vi "excel_read_data.vi"(8 "error in (no error)":errorcluster, 11 "Excel data":path) -> (0 "error out":errorcluster, 2 "wv_length_weight":dbl[](array[numeric]), 3 "wv_length_data":dbl[](array[numeric]))   [LabVIEW 2017]
uses:
  <vilib>/addons/_office/excel.llb/Excel Get Data ([dbl]).vi
  <vilib>/Utility/NIReport.llb/NI_report.lvclass
  <vilib>/Utility/NIReport.llb/Excel/NI_Excel.lvclass
  <vilib>/addons/_office/NI_ReportGenerationToolkit.lvlib
panel:
  out "wv_length and weight":dbl[][](array[numeric]) format="%.2f"
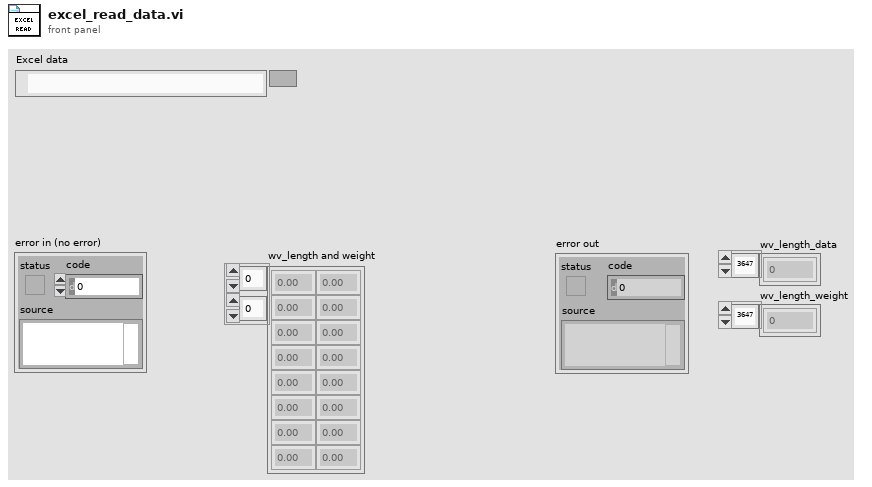
[diagram p1: front panel]
types:
  T1 = enum16{"Standard Report", "HTML", "Word", "Excel"}
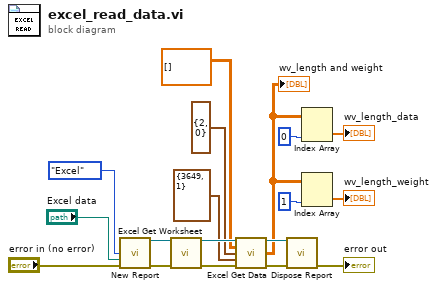
[diagram p0: block diagram]
diagram:
  n1 = call <vilib>:"New Report.vi"("report type"=T1."Excel", "template (empty)"="Excel data", "error in (no error)"="error in (no error)") -> ("report out"=w16:refnum<class "NI_report.lvclass">, "error out"=w15:errorcluster)  [unwired: 11 in]
  n2 = call <vilib>:"Excel Get Worksheet.vi"("report in"=w16, "error in (no error)"=w15) -> ("report out"=w13:refnum<class "NI_report.lvclass">, "error out"=w12:errorcluster)  [unwired: 12 in]
  n3 = call-poly <vilib>:"Excel Get Data.vi"("report in"=w13, "data type"=dbl[][] [], "start (-1, -1)"=cluster{i32, i32} {2, 0}, "end (-1, -1)"=cluster{i32, i32} {3649, 1}, "error in (no error)"=w12) -> ("report out"=w8:refnum<class "NI_report.lvclass">, "data"=w4:dbl[][], "error out"=w7:errorcluster)  [unwired: 8 in]
  "wv_length and weight" <- w4
  n4 = call-dynamic "Dispose Report.vi"("report in"=w8, "error in (no error)"=w7) -> ("error out"=→"error out":errorcluster)  [unwired: 13 in]
  n5 = Index Array(array=w4, index (col)=0 ("disabled index (col)")) -> (element=→"wv_length_data":dbl[])  [unwired: 1 in]
  n6 = Index Array(array=w4, index (col)=1 ("disabled index (col)")) -> (element=→"wv_length_weight":dbl[])  [unwired: 1 in]
